vi "play-with-variants_read_from_file.vi"() -> ()   [LabVIEW 2019]
uses:
  <vilib>/Utility/Data Type/NI_Data Type.lvlib
  <vilib>/Rock Robotics/WPI/ThirdParty/JAS_Junk/TrajLib/TRAJ_CONSTRAINT_CENTRIPETAL_ACCEL.ctl
  <vilib>/Rock Robotics/WPI/ThirdParty/JAS_Junk/TrajLib/Trajectory_Library.lvlib
  <vilib>/Rock Robotics/WPI/ThirdParty/JAS_Junk/TrajLib/DIFF_DRIVE_KINEMATICS.ctl
  <vilib>/Rock Robotics/WPI/ThirdParty/JAS_Junk/TrajLib/TRAJ_CONSTRAINT_DIIF_DRIVE_KINEMATICS.ctl
  <vilib>/Rock Robotics/WPI/ThirdParty/JAS_Junk/TrajLib/TRANSLATION2D.ctl
  <vilib>/Analysis/Matrix/Datatypes/RealMatrix.ctl
  <vilib>/Analysis/Matrix/NI_Matrix.lvlib
  <vilib>/Rock Robotics/WPI/ThirdParty/JAS_Junk/TrajLib/MECA_DRIVE_KINEMATICS.ctl
  <vilib>/Rock Robotics/WPI/ThirdParty/JAS_Junk/TrajLib/TRAJ_CONSTRAINT_MECA_DRIVE_KINEMATICS.ctl
  <vilib>/Rock Robotics/WPI/ThirdParty/JAS_Junk/TrajLib/SWERVE_DRIVE_KINEMATICS.ctl
  <vilib>/Rock Robotics/WPI/ThirdParty/JAS_Junk/TrajLib/TRAJ_CONSTRAINT_SWERVE_DRIVE_KINEMATICS.ctl
  <vilib>/Rock Robotics/WPI/ThirdParty/JAS_Junk/TrajLib/SIMPLE_MOTOR_FF.ctl
  <vilib>/Rock Robotics/WPI/ThirdParty/JAS_Junk/TrajLib/TRAJ_CONSTRAINT_DIIF_DRIVE_VOLTAGE.ctl
  TrajConfig_XML_V5.ctl
  <vilib>/Rock Robotics/WPI/ThirdParty/JAS_Junk/TrajLib/TRAJ_CONFIG.ctl
  <vilib>/Utility/Data Type/Type Definitions/Data Type.ctl
  <vilib>/Utility/Data Type/Type Definitions/Type Definition Info.ctl
panel:
  out "value":T1 {"CentAccelConstraint"."Max Cent Accel" format="%20.4f"; "DiffDriveKineConstraint"."Max Accel (M/S2)" format="%20.4f"; "DiffDriveKineConstraint"."DIFF_DRIVE_KINEMATICS"."TrackWidth_Meters" format="%20.4f"; "DiffDriveKineConstraint"."Max Speed (M/S)" format="%20.4f"; "MecaKineConstraint"."MECA_DRIVE_KINEMATICS"."PrevCoR"."Y" format="%14.3f"; "MecaKineConstraint"."MECA_DRIVE_KINEMATICS"."PrevCoR"."X" format="%14.3f"; "MecaKineConstraint"."MECA_DRIVE_KINEMATICS"."RearRight"."Y" format="%14.3f"; "MecaKineConstraint"."MECA_DRIVE_KINEMATICS"."RearRight"."X" format="%14.3f"; "MecaKineConstraint"."MECA_DRIVE_KINEMATICS"."RearLeft"."Y" format="%14.3f"; "MecaKineConstraint"."MECA_DRIVE_KINEMATICS"."RearLeft"."X" format="%14.3f"; "MecaKineConstraint"."MECA_DRIVE_KINEMATICS"."FrontRight"."Y" format="%14.3f"; "MecaKineConstraint"."MECA_DRIVE_KINEMATICS"."FrontRight"."X" format="%14.3f"; "MecaKineConstraint"."MECA_DRIVE_KINEMATICS"."FrontLeft"."Y" format="%14.3f"; "MecaKineConstraint"."MECA_DRIVE_KINEMATICS"."FrontLeft"."X" format="%14.3f"; "MecaKineConstraint"."Max Speed (M/S)" format="%20.4f"; "SwerveKineConstraint"."SwerveKinematics"."PrevCoR"."Y" format="%14.3f"; "SwerveKineConstraint"."SwerveKinematics"."PrevCoR"."X" format="%14.3f"; "SwerveKineConstraint"."SwerveKinematics"."Modules"."Y" format="%14.3f"; "SwerveKineConstraint"."SwerveKinematics"."Modules"."X" format="%14.3f"; "SwerveKineConstraint"."Max Speed (M/S)" format="%20.4f"; "DiffVoltConstraint"."SIMPLE_MOTOR_FF"."Ka" format="%13.4f"; "DiffVoltConstraint"."SIMPLE_MOTOR_FF"."Kv" format="%13.4f"; "DiffVoltConstraint"."SIMPLE_MOTOR_FF"."Ks" format="%13.4f"; "DiffVoltConstraint"."DIFF_DRIVE_KINEMATICS"."TrackWidth_Meters" format="%20.4f"; "DiffVoltConstraint"."Max Voltage" format="%20.4f"}
  out "error out 2":errorcluster
  out "text":string
  out "error out":errorcluster
  out "Constraints":variant[](array[variant])
  out "TypeDefInfo":T13[](array[typedef])
  out "TypeDef":bool[](array[boolean])
  out "Name":string[](array[string])
  out "Type":T14[](array[typedef])
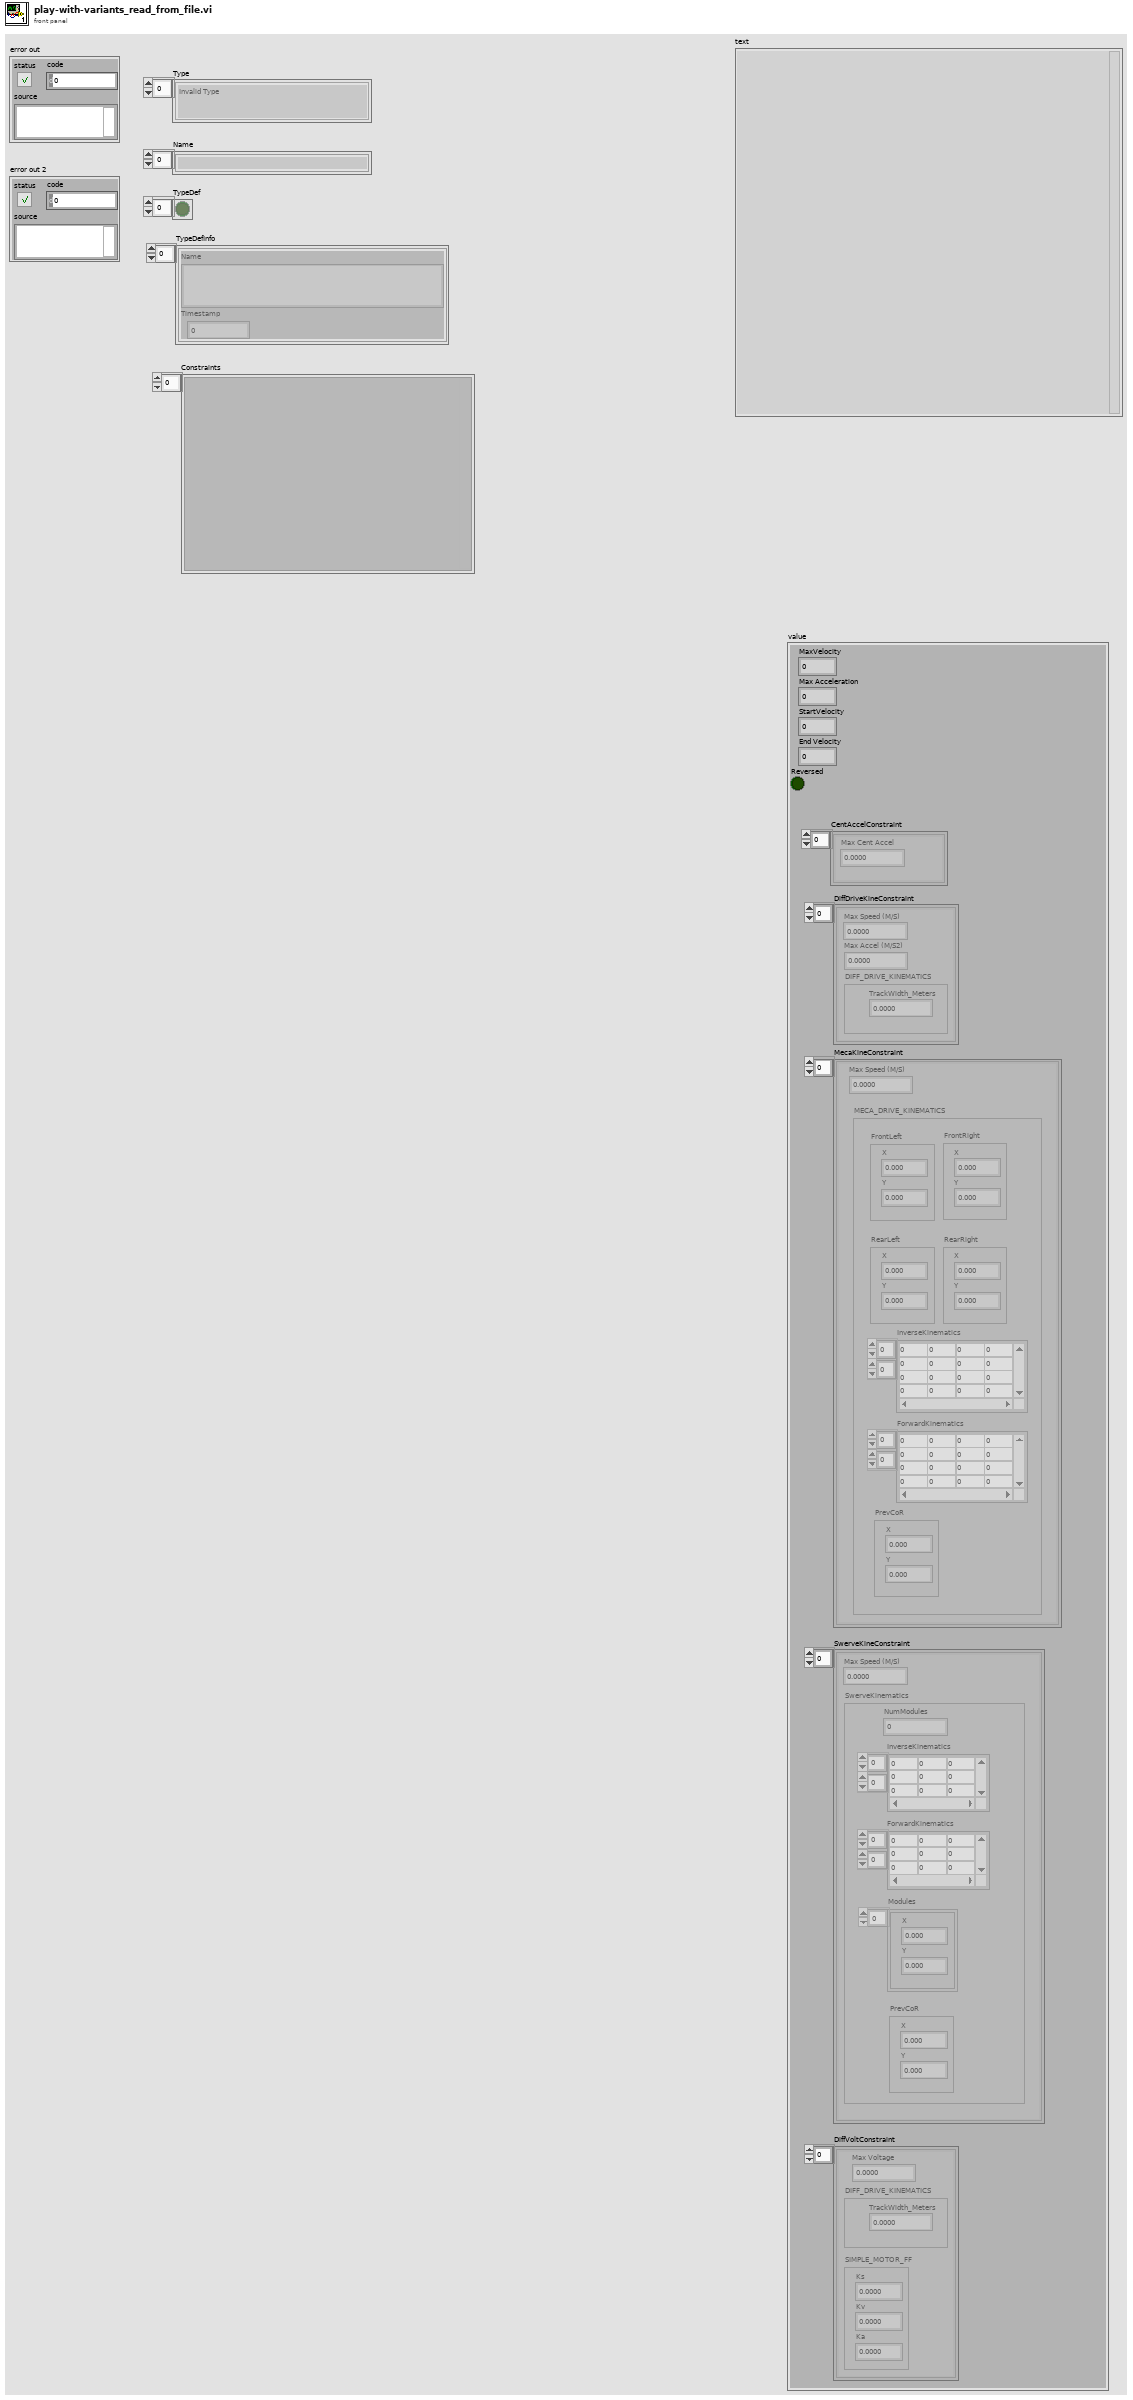
[diagram p1: front panel]
types:
  T1 = typedef "TrajConfig_XML_V5.ctl" = cluster{"MaxVelocity":dbl, "Max Acceleration":dbl, "StartVelocity":dbl, "End Velocity":dbl, "Reversed":bool, "CentAccelConstraint":T2[], "DiffDriveKineConstraint":T3[], "MecaKineConstraint":T5[], "SwerveKineConstraint":T9[], "DiffVoltConstraint":T11[]}
  T2 = typedef "Trajectory_Library.lvlib/TRAJ_CONSTRAINT_CENTRIPETAL_ACCEL.ctl" = cluster{"Max Cent Accel":dbl}
  T3 = typedef "Trajectory_Library.lvlib/TRAJ_CONSTRAINT_DIIF_DRIVE_KINEMATICS.ctl" = cluster{"Max Speed (M/S)":dbl, "DIFF_DRIVE_KINEMATICS":T4, "Max Accel (M/S2)":dbl}
  T4 = typedef "Trajectory_Library.lvlib/DIFF_DRIVE_KINEMATICS.ctl" = cluster{"TrackWidth_Meters":dbl}
  T5 = typedef "Trajectory_Library.lvlib/TRAJ_CONSTRAINT_MECA_DRIVE_KINEMATICS.ctl" = cluster{"Max Speed (M/S)":dbl, "MECA_DRIVE_KINEMATICS":T6}
  T6 = typedef "Trajectory_Library.lvlib/MECA_DRIVE_KINEMATICS.ctl" = cluster{"FrontLeft":T7, "FrontRight":T7, "RearLeft":T7, "RearRight":T7, "InverseKinematics":T8, "ForwardKinematics":T8, "PrevCoR":T7}
  T7 = typedef "Trajectory_Library.lvlib/TRANSLATION2D.ctl" = cluster{"X":dbl, "Y":dbl}
  T8 = typedef "NI_Matrix.lvlib/RealMatrix.ctl" = dbl[][]
  T9 = typedef "Trajectory_Library.lvlib/TRAJ_CONSTRAINT_SWERVE_DRIVE_KINEMATICS.ctl" = cluster{"Max Speed (M/S)":dbl, "SwerveKinematics":T10}
  T10 = typedef "Trajectory_Library.lvlib/SWERVE_DRIVE_KINEMATICS.ctl" = cluster{"NumModules":i32, "InverseKinematics":T8, "ForwardKinematics":T8, "Modules":T7[], "PrevCoR":T7}
  T11 = typedef "Trajectory_Library.lvlib/TRAJ_CONSTRAINT_DIIF_DRIVE_VOLTAGE.ctl" = cluster{"Max Voltage":dbl, "DIFF_DRIVE_KINEMATICS":T4, "SIMPLE_MOTOR_FF":T12}
  T12 = typedef "Trajectory_Library.lvlib/SIMPLE_MOTOR_FF.ctl" = cluster{"Ks":dbl, "Kv":dbl, "Ka":dbl}
  T13 = typedef "NI_Data Type.lvlib/Type Definition Info.ctl" = cluster{"Name":string, "Timestamp":u32}
  T14 = typedef "NI_Data Type.lvlib/Data Type.ctl" = enum8{"Invalid Type", "Void", "I8", "I16", "I32", "I64", "U8", "U16", "U32", "U64", "Single Float", "Double Float", "Extended Float", "Single Complex", "Double Complex", "Extended Complex", "Enum U8", "Enum U16", "Enum U32", "Enum U64", "Single Float With Unit", "Double Float With Unit", "Extended Float With Unit", "Single Complex with Unit", "Double Complex with Unit", "Extended Complex with Unit", "Boolean", "String", "Path", "Picture", "Tag", "Array", "Cluster", "Variant", "LV Variant", "Waveform", "Timestamp", "Digital Waveform", "Digital Data", "ExpressData", "Refnum", "External Data", "VI", "Poly VI", "LabVIEW Class Instance", "Fixed Point", "Set Collection", "Map Collection"}
  T15 = typedef "Trajectory_Library.lvlib/TRAJ_CONFIG.ctl" = cluster{"MaxVelocity":dbl, "Max Acceleration":dbl, "StartVelocity":dbl, "End Velocity":dbl, "Reversed":bool, "Constraints":variant[]}
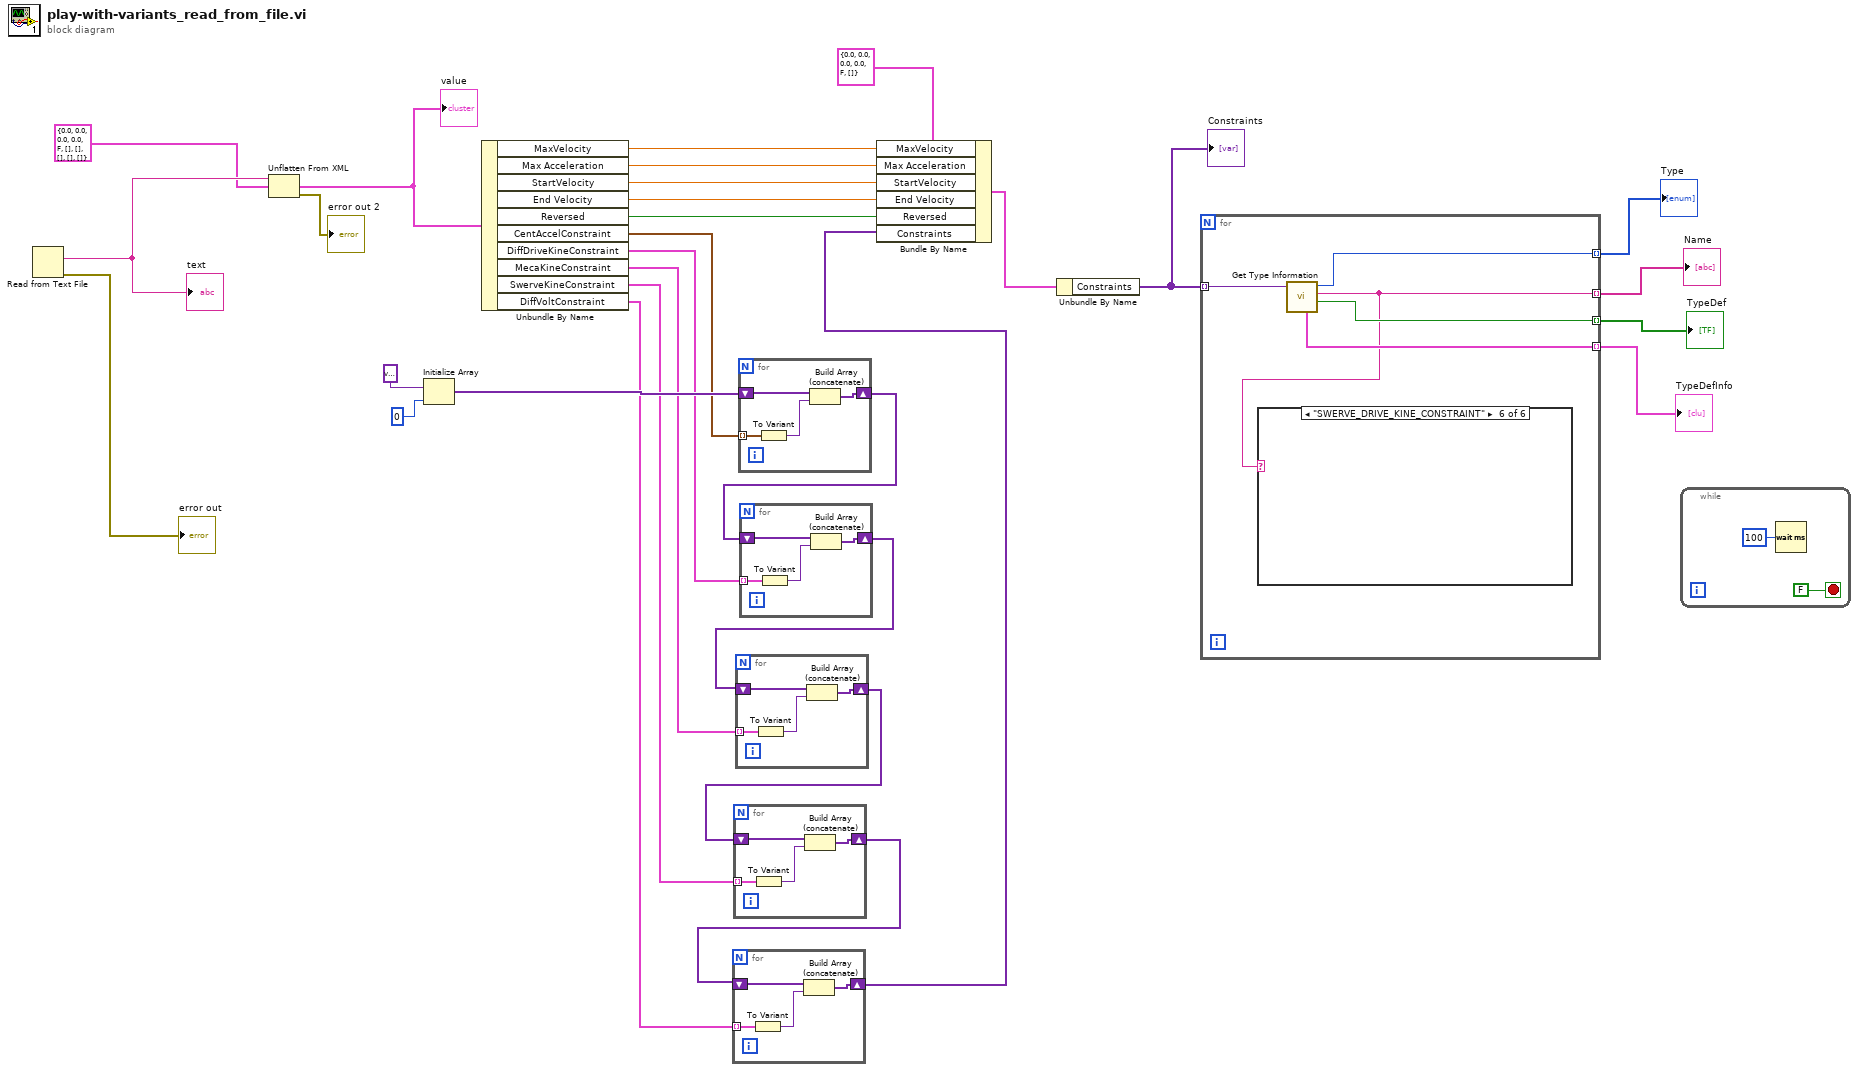
[diagram p0: block diagram]
diagram:
  n1 = Read from Text File() -> (text=w23:string, error out=→"error out":errorcluster)  [unwired: 4 in, 2 out]
  "text" <- w23
  n2 = Unflatten From XML(xml string=w23, type=T1 {"MaxVelocity"=0.0, "Max Acceleration"=0.0, "StartVelocity"=0.0, "End Velocity"=0.0, "Reversed"=FALSE, "CentAccelConstraint"=[], "DiffDriveKineConstraint"=[], "MecaKineConstraint"=[], "SwerveKineConstraint"=[], "DiffVoltConstraint"=[]} ("TrajConfigXML_V5")) -> (value=w21:T1, error out=→"error out 2":errorcluster)  [unwired: 1 in]
  "value" <- w21
  n3 = Initialize Array(variant, 0 ("dimension size")) -> (w11:variant[])
  n4 = Unbundle By Name(w21) -> ("MaxVelocity"=w19:dbl, "Max Acceleration"=w17:dbl, "StartVelocity"=w16:dbl, "End Velocity"=w15:dbl, "Reversed"=w14:bool, "CentAccelConstraint"=w10:T2[], "DiffDriveKineConstraint"=w3:T3[], "MecaKineConstraint"=w4:T5[], "SwerveKineConstraint"=w2:T9[], "DiffVoltConstraint"=w1:T11[])
  n5 = for {
    shift-right: [w32] -> w9
    shift-left: w11 -> [w34]
    tunnel: w10 -> [w31] mode=indexing
    n6 = To Variant(anything=w31) -> (Variant=w33:variant)
    n7 = Build Array (concatenate)(w34, w33) -> (w32:variant[])
  }
  n8 = for {
    shift-right: [w36] -> w8
    shift-left: w9 -> [w38]
    tunnel: w3 -> [w35] mode=indexing
    n9 = To Variant(anything=w35) -> (Variant=w37:variant)
    n10 = Build Array (concatenate)(w38, w37) -> (w36:variant[])
  }
  n11 = for {
    shift-right: [w40] -> w7
    shift-left: w8 -> [w42]
    tunnel: w4 -> [w39] mode=indexing
    n12 = To Variant(anything=w39) -> (Variant=w41:variant)
    n13 = Build Array (concatenate)(w42, w41) -> (w40:variant[])
  }
  n14 = for {
    shift-right: [w44] -> w6
    shift-left: w7 -> [w46]
    tunnel: w2 -> [w43] mode=indexing
    n15 = To Variant(anything=w43) -> (Variant=w45:variant)
    n16 = Build Array (concatenate)(w46, w45) -> (w44:variant[])
  }
  n17 = for {
    shift-right: [w48] -> w5
    shift-left: w6 -> [w50]
    tunnel: w1 -> [w47] mode=indexing
    n18 = To Variant(anything=w47) -> (Variant=w49:variant)
    n19 = Build Array (concatenate)(w50, w49) -> (w48:variant[])
  }
  n20 = Bundle By Name(cluster=T15 {"MaxVelocity"=0.0, "Max Acceleration"=0.0, "StartVelocity"=0.0, "End Velocity"=0.0, "Reversed"=FALSE, "Constraints"=[]} ("TRAJECTORY_CONFIG"), "MaxVelocity"=w19, "Max Acceleration"=w17, "StartVelocity"=w16, "End Velocity"=w15, "Reversed"=w14, "Constraints"=w5) -> (w18:T15)
  n21 = Unbundle By Name(w18) -> ("Constraints"=w26:variant[])
  "Constraints" <- w26
  n22 = for {
    tunnel: [w55] -> w30 mode=indexing
    tunnel: [w52] -> w29 mode=indexing
    tunnel: [w53] -> w28 mode=indexing
    tunnel: [w54] -> w27 mode=indexing
    tunnel: w26 -> [w51] mode=indexing
    n23 = call <vilib>:"Get Type Information.vi"("variant"=w51) -> ("type definition"=w53:bool, "name"=w52:string, "type"=w55:T14, "type definition info"=w54:T13)  [unwired: 6 in, 1 out]
    n24 = case shown="\"SWERVE_DRIVE_KINE_CONSTRAINT\"" w52 {
      frame Default {
      }
      frame "DIFF_DRIVE_KINE_CONSTRAINT" {
      }
      frame "CENTRIPETAL_ACCEL_CONSTRAINT" {
      }
      frame "DIFF_DRIVE_VOLTAGE_CONSTRAINT" {
      }
      frame "MECANUM_DRIVE_KINE_CONSTRAINT" {
      }
      frame "SWERVE_DRIVE_KINE_CONSTRAINT" {
      }
    }
  }
  "Type" <- w30
  "Name" <- w29
  "TypeDef" <- w28
  "TypeDefInfo" <- w27
  n25 = while {
    stop <- FALSE stop-if-true
    n26 = Wait (ms)(milliseconds to wait=u32 100) -> ()  [unwired: 1 out]
  }
